vi "SV Data Type.vi"(8 "Error In":errorcluster, 11 "Data Type - Variant":variant[](array[variant])) -> (0 "Error Out":errorcluster, 2 "Type array":string[](array[string]), 3 "no. variables":i32)   [LabVIEW 2014]
doc: "<B>Copyright</B>: (c) 2015 MHWirth. All rights reserved.\n\nThis VI recieves an array of variants and specifies the data type associated to every variant. \n\nIf a type is not supported, it returns \"Not Known Data Type\".\n\nThe supported data types are\n- String\n- Boolean\n- Int8, Int16, Int32, Int64\n- UInt8, UInt16, UInt32, UInt64\n- Single-precision\n- Double\n- Fixed Point - signed\n- Fixed Point - unsigned\n- 1D array of (Boolean, Int8, Int16, ...)\n- 2D array of (Boolean, Int8, Int16, ...)\n\n<B>Error 7000</B> Undefined SV Data Type"
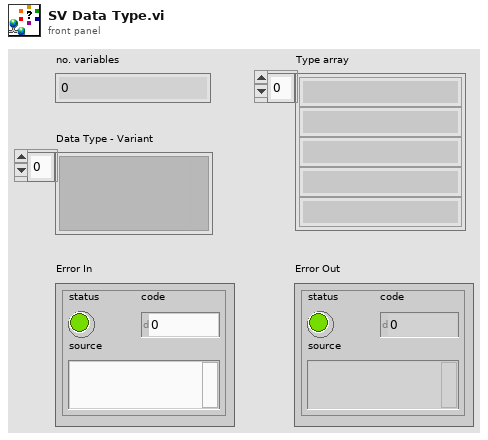
[diagram p1: front panel]
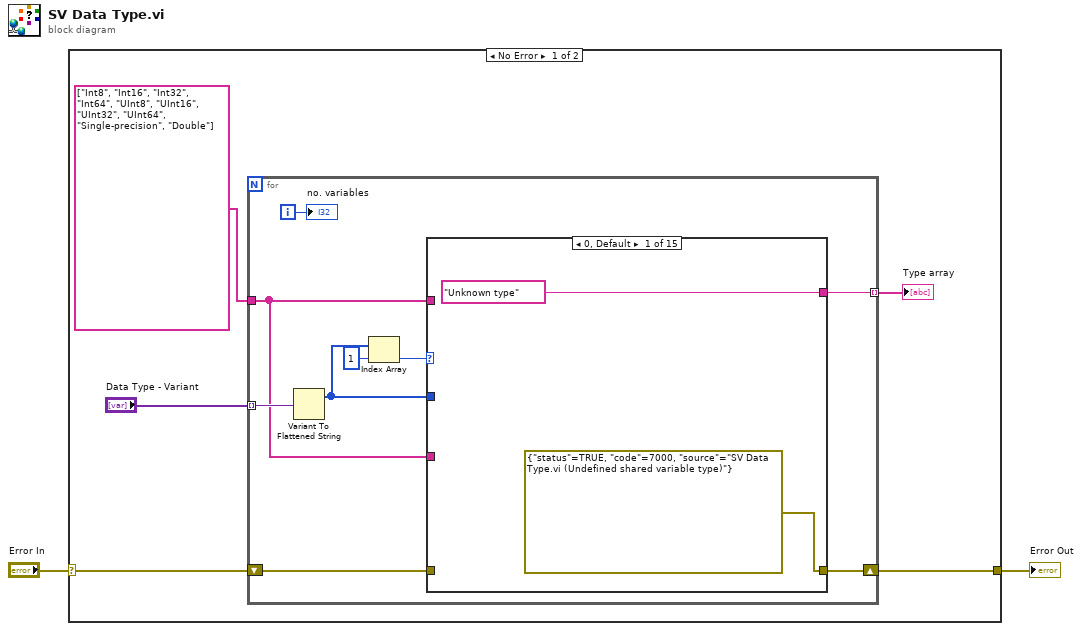
[diagram p0: block diagram]
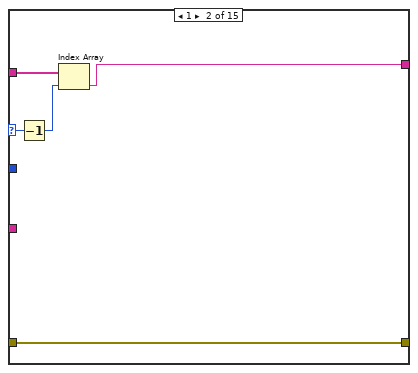
[diagram p2: hidden frame]
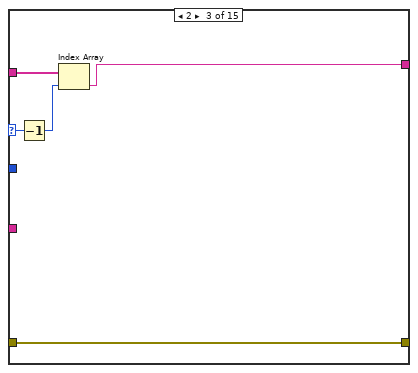
[diagram p3: hidden frame]
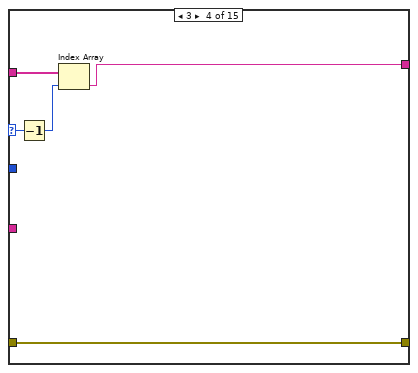
[diagram p4: hidden frame]
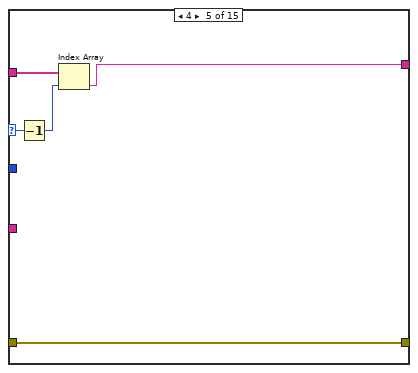
[diagram p5: hidden frame]
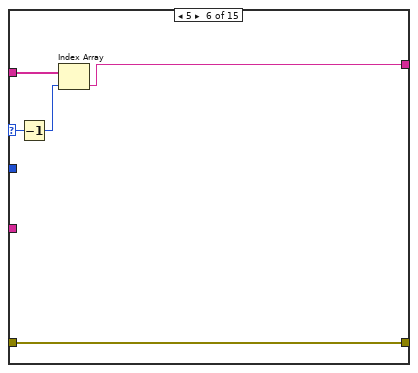
[diagram p6: hidden frame]
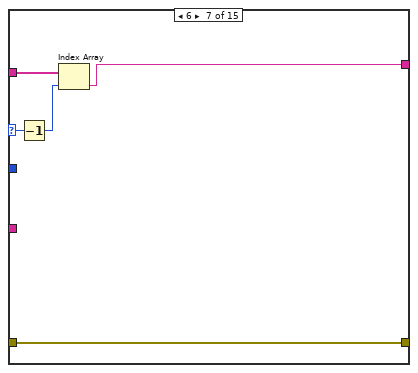
[diagram p7: hidden frame]
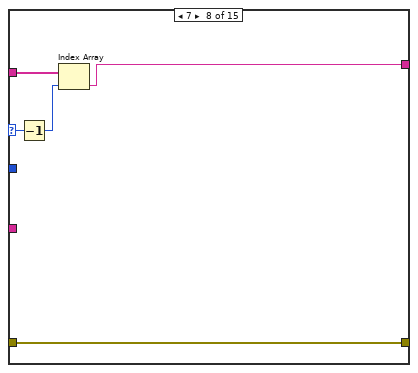
[diagram p8: hidden frame]
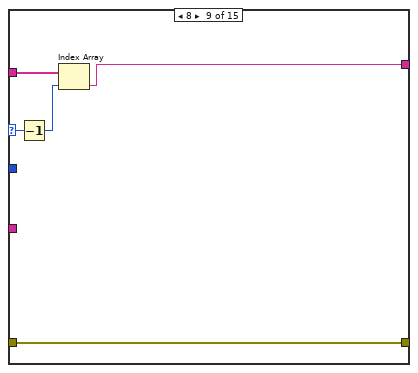
[diagram p9: hidden frame]
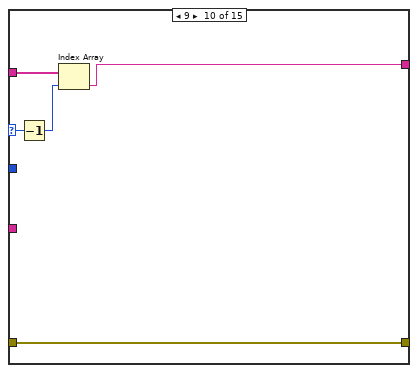
[diagram p10: hidden frame]
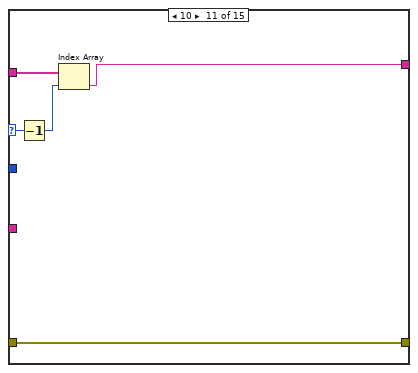
[diagram p11: hidden frame]
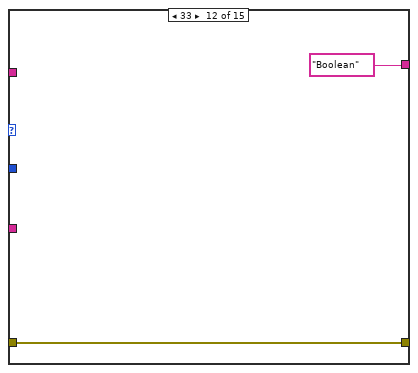
[diagram p12: hidden frame]
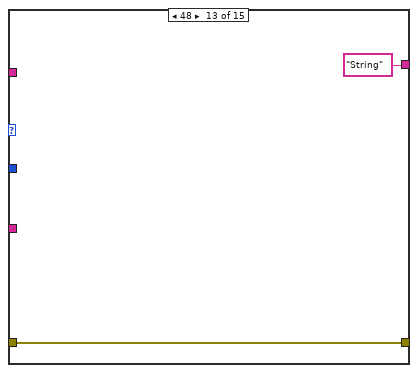
[diagram p13: hidden frame]
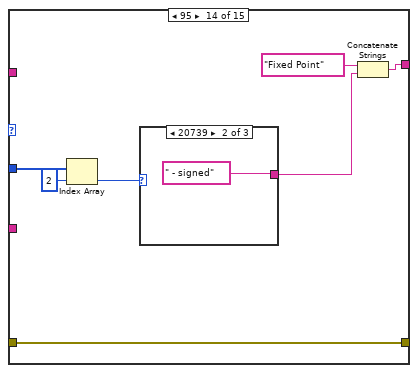
[diagram p14: hidden frame]
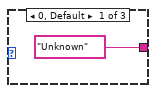
[diagram p15: hidden frame]
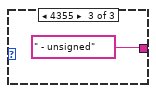
[diagram p16: hidden frame]
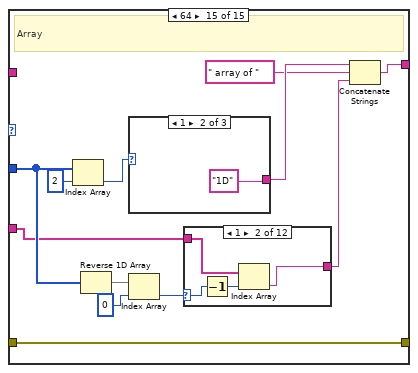
[diagram p17: hidden frame]
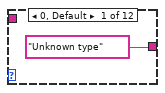
[diagram p18: hidden frame]
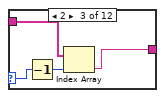
[diagram p19: hidden frame]
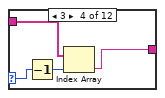
[diagram p20: hidden frame]
diagram:
  n1 = case shown="No Error" "Error In" {
    selector: "Error In" -> [w6 w140]
    tunnel: [w5 w140] -> w1
    frame No Error {
      n2 = for {
        tunnel: "Data Type - Variant" -> [w15] mode=indexing
        shift-right: [w8] -> w5
        shift-left: w6 -> [w9]
        tunnel: string[] ["Int8", "Int16", "Int32", "Int64", "UInt8", "UInt16", "UInt32", "UInt64", "Single-precision", "Double"] -> [w11]
        tunnel: [w12] -> w3 mode=indexing
        i -> [w16]
        n3 = Variant To Flattened String(Variant=w15) -> (1:w10:i16[])  [unwired: 1 out]
        n4 = Index Array(array=w10, index=1) -> (element=w13:i16)
        n5 = case shown="0, Default" w13 {
          selector: w13 -> [_ w21 w26 w31 w36 w41 w46 w51 w56 w61 w66 _ _ _ _]
          tunnel: ["Unknown type" w22 w27 w32 w37 w42 w47 w52 w57 w62 w67 "Boolean" "String" w75 w87] -> w12
          tunnel: w11 -> [_ w23 w28 w33 w38 w43 w48 w53 w58 w63 w68 _ _ _ _]
          tunnel: w10 -> [_ _ _ _ _ _ _ _ _ _ _ _ _ w79 w92]
          tunnel: w11 -> [_ _ _ _ _ _ _ _ _ _ _ _ _ _ w86]
          tunnel: w9 -> [_ w19 w24 w29 w34 w39 w44 w49 w54 w59 w64 w69 w71 w73 w83]
          tunnel: [errorcluster {"status"=TRUE, "code"=7000, "source"="SV Data Type.vi (Undefined shared variable type)"} ("error IO") w19 w24 w29 w34 w39 w44 w49 w54 w59 w64 w69 w71 w73 w83] -> w8
          frame 0, Default {
          }
          frame 1 {
            n6 = Decrement(x=w21) -> (x-1=w20:i16)
            n7 = Index Array(array=w23, index=w20) -> (element=w22:string)
          }
          frame 2 {
            n8 = Decrement(x=w26) -> (x-1=w25:i16)
            n9 = Index Array(array=w28, index=w25) -> (element=w27:string)
          }
          frame 3 {
            n10 = Decrement(x=w31) -> (x-1=w30:i16)
            n11 = Index Array(array=w33, index=w30) -> (element=w32:string)
          }
          frame 4 {
            n12 = Decrement(x=w36) -> (x-1=w35:i16)
            n13 = Index Array(array=w38, index=w35) -> (element=w37:string)
          }
          frame 5 {
            n14 = Decrement(x=w41) -> (x-1=w40:i16)
            n15 = Index Array(array=w43, index=w40) -> (element=w42:string)
          }
          frame 6 {
            n16 = Decrement(x=w46) -> (x-1=w45:i16)
            n17 = Index Array(array=w48, index=w45) -> (element=w47:string)
          }
          frame 7 {
            n18 = Decrement(x=w51) -> (x-1=w50:i16)
            n19 = Index Array(array=w53, index=w50) -> (element=w52:string)
          }
          frame 8 {
            n20 = Decrement(x=w56) -> (x-1=w55:i16)
            n21 = Index Array(array=w58, index=w55) -> (element=w57:string)
          }
          frame 9 {
            n22 = Decrement(x=w61) -> (x-1=w60:i16)
            n23 = Index Array(array=w63, index=w60) -> (element=w62:string)
          }
          frame 10 {
            n24 = Decrement(x=w66) -> (x-1=w65:i16)
            n25 = Index Array(array=w68, index=w65) -> (element=w67:string)
          }
          frame 33 {
          }
          frame 48 {
          }
          frame 95 {
            n26 = Index Array(array=w79, index=2) -> (element=w77:i16)
            n27 = case shown="20739" w77 {
              tunnel: ["Unknown" " - signed" " - unsigned"] -> w74
              frame 0, Default {
              }
              frame 20739 {
              }
              frame 4355 {
              }
            }
            n28 = Concatenate Strings("Fixed Point", w74) -> (w75:string)
          }
          frame 64 {
            # "Array"
            n29 = Index Array(array=w92, index=2) -> (element=w93:i16)
            n30 = Reverse 1D Array(array=w92) -> (reversed array=w91:i16[])
            n31 = case shown="1" w93 {
              tunnel: ["Unknown dim" "1D" "2D"] -> w89
              frame 0, Default {
              }
              frame 1 {
              }
              frame 2 {
              }
            }
            n32 = Index Array(array=w91, index=0) -> (element=w85:i16)
            n33 = case shown="1" w85 {
              selector: w85 -> [_ w99 w103 w107 w111 w115 w119 w123 w127 w131 w135 _]
              tunnel: w86 -> [_ w97 w101 w105 w109 w113 w117 w121 w125 w129 w133 _]
              tunnel: ["Unknown type" w96 w100 w104 w108 w112 w116 w120 w124 w128 w132 "Boolean"] -> w84
              frame 0, Default {
              }
              frame 1 {
                n34 = Decrement(x=w99) -> (x-1=w98:i16)
                n35 = Index Array(array=w97, index=w98) -> (element=w96:string)
              }
              frame 2 {
                n36 = Decrement(x=w103) -> (x-1=w102:i16)
                n37 = Index Array(array=w101, index=w102) -> (element=w100:string)
              }
              frame 3 {
                n38 = Decrement(x=w107) -> (x-1=w106:i16)
                n39 = Index Array(array=w105, index=w106) -> (element=w104:string)
              }
              frame 4 {
                n40 = Decrement(x=w111) -> (x-1=w110:i16)
                n41 = Index Array(array=w109, index=w110) -> (element=w108:string)
              }
              frame 5 {
                n42 = Decrement(x=w115) -> (x-1=w114:i16)
                n43 = Index Array(array=w113, index=w114) -> (element=w112:string)
              }
              frame 6 {
                n44 = Decrement(x=w119) -> (x-1=w118:i16)
                n45 = Index Array(array=w117, index=w118) -> (element=w116:string)
              }
              frame 7 {
                n46 = Decrement(x=w123) -> (x-1=w122:i16)
                n47 = Index Array(array=w121, index=w122) -> (element=w120:string)
              }
              frame 8 {
                n48 = Decrement(x=w127) -> (x-1=w126:i16)
                n49 = Index Array(array=w125, index=w126) -> (element=w124:string)
              }
              frame 9 {
                n50 = Decrement(x=w131) -> (x-1=w130:i16)
                n51 = Index Array(array=w129, index=w130) -> (element=w128:string)
              }
              frame 10 {
                n52 = Decrement(x=w135) -> (x-1=w134:i16)
                n53 = Index Array(array=w133, index=w134) -> (element=w132:string)
              }
              frame 33 {
              }
            }
            n54 = Concatenate Strings(w89, " array of ", w84) -> (w87:string)
          }
        }
        "no. variables" <- w16
      }
      "Type array" <- w3
    }
    frame Error {
    }
  }
  "Error Out" <- w1
